vi "Global Vars.vi"() -> ()   [LabVIEW 2012]
panel:
  out "Z Pos":dbl
  out "Pause XY-4":bool
  out "Pause CPMG":bool
  out "Pause SpinEcho":bool
  out "Pause Rabi":bool
  out "XY4-ing":bool
  out "CPMG-ing":bool
  out "Stability-ing":bool
  out "Spectrum-ing":bool
  out "SpinEcho-ing":bool
  out "Counts":u32
  out "Rabi-ing":bool
  out "ESR-ing":bool
  out "Counting":bool
  out "Optimizing":bool
  out "Scanning":bool
  out "Y Pos":dbl
  out "X Pos":dbl
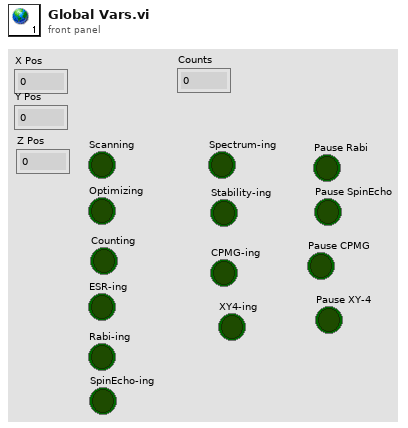
[diagram p1: front panel]
diagram:
